vi "Vending Machine.vi"() -> ()   [LabVIEW 2020]
uses:
  Case Selector.ctl
panel:
  out "Current Money":dbl
  out "Change":dbl
  out "Product Delivered":bool
  in  "Insert Coins":cluster{"5 Cents":bool, "10 Cents":bool}
  in  "Choose from \nthese:":T1
  in  "Stop":bool
  # "Price Per Item"
  # "Add Money Here"
  # "60 cents"
  # "75 cents"
  # "60 cents"
  # "75 cents"
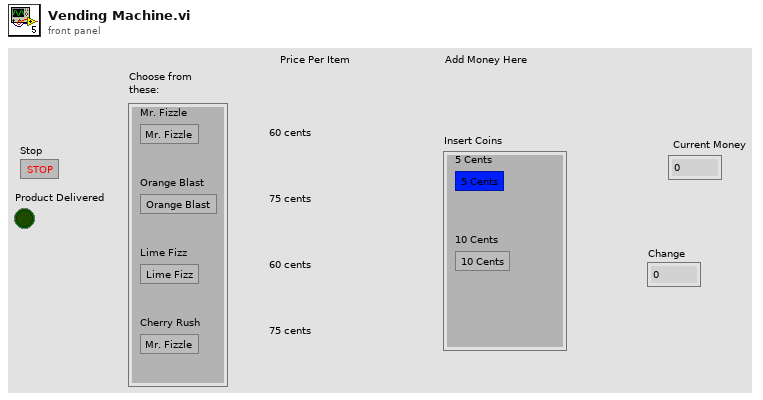
[diagram p1: front panel]
types:
  T1 = cluster{"Mr. Fizzle":bool, "Orange Blast":bool, "Lime Fizz":bool, "Cherry Rush":bool}
  T2 = typedef "Case Selector.ctl" = enum16{"Return Change", "Select Product", "Add Money", "Waiting", "Start-Up", "Dispense Product"}
  T3 = enum16{"Return Change", "Select Product", "Add Money", "Waiting", "Start-Up"}
  T4 = cluster{"Cherry Rush":bool, "Lime Fizz":bool, "Orange Blast":bool, "Mr. Fizzle":bool}
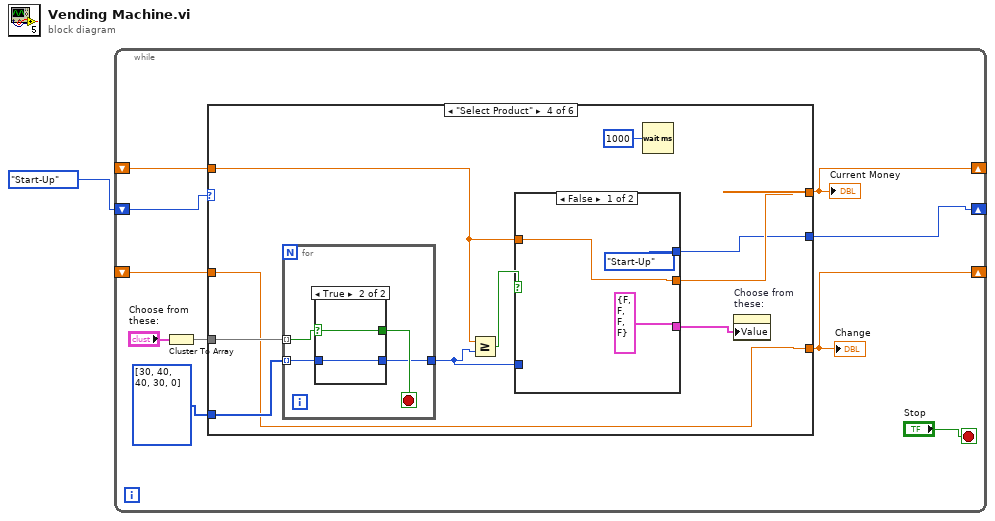
[diagram p0: block diagram]
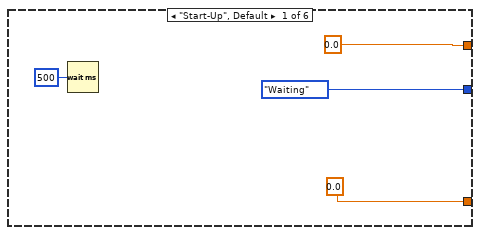
[diagram p2: hidden frame]
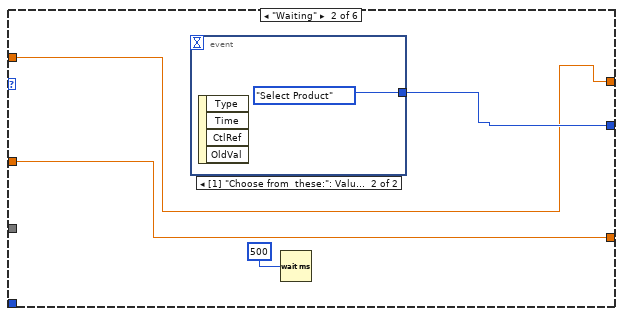
[diagram p3: hidden frame]
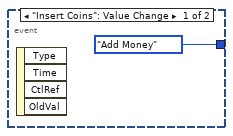
[diagram p4: hidden frame]
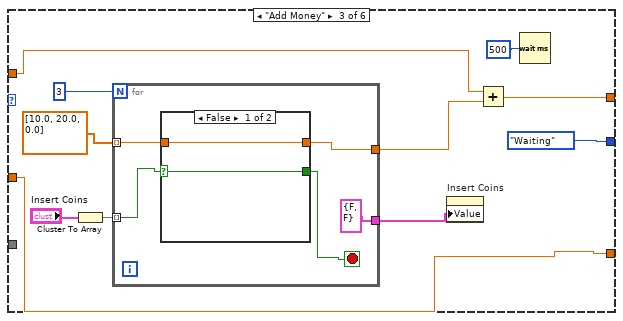
[diagram p5: hidden frame]
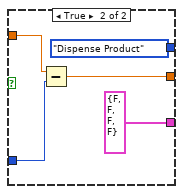
[diagram p7: hidden frame]
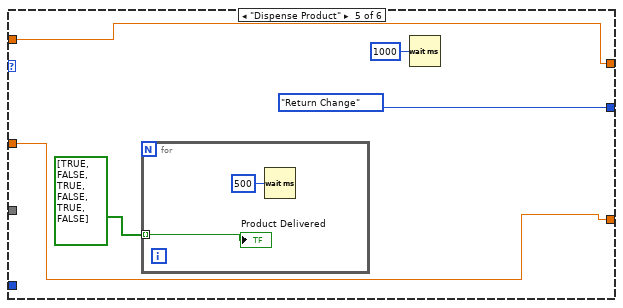
[diagram p9: hidden frame]
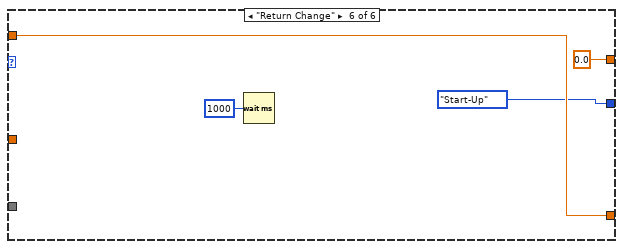
[diagram p10: hidden frame]
diagram:
  n1 = while {
    shift-right: [w10] -> _
    shift-left: Case_Selector."Start-Up" ("Enum") -> [w11]
    shift-right: [w5] -> _
    shift-left: _ -> [w6]
    shift-right: [w4] -> _
    shift-left: _ -> [w3]
    stop <- "Stop" stop-if-true
    n2 = Cluster To Array(cluster="Choose from \nthese:") -> (array=w8:bool[])
    n3 = case shown="\"Select Product\"" w11 {
      tunnel: [T3."Waiting" ("Enum") w19 Case_Selector."Waiting" ("Enum") w45 Case_Selector."Return Change" ("Enum") Case_Selector."Start-Up" ("Enum")] -> w10
      tunnel: [0.0 w17 w26 w46 w72 0.0] -> w5
      tunnel: w8 -> [_ _ _ w51 _ _]
      tunnel: i32[] [30, 40, 40, 30, 0] -> [_ _ _ w50 _ _]
      tunnel: w6 -> [_ w17 w24 w47 w72 w77]
      tunnel: [0.0 w18 w27 w44 w70 w77] -> w4
      tunnel: w3 -> [_ w18 w27 w44 w70 _]
      frame "Start-Up", Default {
        n4 = Wait (ms)(milliseconds to wait=u32 500) -> ()  [unwired: 1 out]
      }
      frame "Waiting" {
        n5 = event shown="[1] \"Choose from  these:\": Value Change" {
          selector: _ -> [_ _]
          dyn-events: _ -> [_ _]
          timeout: _ -> [_ _]
          tunnel: [Case_Selector."Add Money" ("Enum") T3."Select Product" ("Enum")] -> w19
          event "Insert Coins": Value Change {
            n6 = event-data() -> ()  [unwired: 1 in, 4 out]
          }
          event "Choose from \nthese:": Value Change {
            n7 = event-data() -> ()  [unwired: 1 in, 4 out]
          }
        }
        n8 = Wait (ms)(milliseconds to wait=u32 500) -> ()  [unwired: 1 out]
      }
      frame "Add Money" {
        n9 = Cluster To Array(cluster="Insert Coins") -> (array=w30:bool[])
        n10 = for {
          N: 3 -> [_]
          tunnel: w30 -> [w37] mode=indexing
          tunnel: dbl[] [10.0, 20.0, 0.0] -> [w36] mode=indexing
          tunnel: [w35] -> w25
          tunnel: [cluster{"10 Cents":bool, "5 Cents":bool} {"10 Cents"=FALSE, "5 Cents"=FALSE} ("Insert Coins")] -> w23
          stop <- w33 stop-if-true
          n11 = case shown="False" w37 {
            selector: w37 -> [w38 w40]
            tunnel: w36 -> [w39 w41]
            tunnel: [w39 w41] -> w35
            tunnel: [w38 w40] -> w33
            frame False {
            }
            frame True {
            }
          }
        }
        n12 = property on="Insert Coins" class="Clust (strict)"("Value"=w23) -> ()  [unwired: 2 in, 2 out]
        n13 = Add(x=w24, y=w25) -> (x+y=w26:dbl)
        n14 = Wait (ms)(milliseconds to wait=u32 500) -> ()  [unwired: 1 out]
      }
      frame "Select Product" {
        n15 = for {
          tunnel: w51 -> [w63] mode=indexing
          tunnel: w50 -> [w61] mode=indexing
          tunnel: [w60] -> w48
          stop <- w62 stop-if-true
          n16 = case shown="True" w63 {
            selector: w63 -> [w65 w67]
            tunnel: [w65 w67] -> w62
            tunnel: w61 -> [w64 w66]
            tunnel: [w64 w66] -> w60
            frame False {
            }
            frame True {
            }
          }
        }
        n17 = Greater Or Equal?(x=w47, y=w48) -> (x >= y?=w49:bool)
        n18 = case shown="False" w49 {
          tunnel: w48 -> [_ w58]
          tunnel: w47 -> [w54 w59]
          tunnel: [w54 w57] -> w46
          tunnel: [Case_Selector."Start-Up" ("Enum") Case_Selector."Dispense Product" ("Enum")] -> w45
          tunnel: [T4 {"Cherry Rush"=FALSE, "Lime Fizz"=FALSE, "Orange Blast"=FALSE, "Mr. Fizzle"=FALSE} ("Choose from \nthese:") T4 {"Cherry Rush"=FALSE, "Lime Fizz"=FALSE, "Orange Blast"=FALSE, "Mr. Fizzle"=FALSE} ("Choose from \nthese:")] -> w42
          frame False {
          }
          frame True {
            n19 = Subtract(x=w59, y=w58) -> (x-y=w57:dbl)
          }
        }
        n20 = Wait (ms)(milliseconds to wait=u32 1000) -> ()  [unwired: 1 out]
        n21 = property on="Choose from \nthese:" class="Clust (strict)"("Value"=w42) -> ()  [unwired: 2 in, 2 out]
      }
      frame "Dispense Product" {
        n22 = for {
          tunnel: bool[] [TRUE, FALSE, TRUE, FALSE, TRUE, FALSE] -> [w73] mode=indexing
          n23 = Wait (ms)(milliseconds to wait=u32 500) -> ()  [unwired: 1 out]
          "Product Delivered" <- w73
        }
        n24 = Wait (ms)(milliseconds to wait=u32 1000) -> ()  [unwired: 1 out]
      }
      frame "Return Change" {
        n25 = Wait (ms)(milliseconds to wait=u32 1000) -> ()  [unwired: 1 out]
      }
    }
    "Current Money" <- w5
    "Change" <- w4
  }
